vi "test_Get Slot.vi"(8 "error in (no error)":errorcluster, 11 "TestCase in":refnum<class "Scan Engine Scripting API Custom Device Unit Tests.lvclass">) -> (0 "error out":errorcluster, 3 "TestCase out":refnum<class "Scan Engine Scripting API Custom Device Unit Tests.lvclass">)   [LabVIEW 2017, in "Scan Engine Scripting API Custom Device Unit Tests.lvclass"]
uses:
  Scan Engine Scripting API Custom Device Unit Tests.lvclass
  Type Defs/Main Settings.ctl
  Type Defs/Local Chassis Settings.ctl
  Scan Engine Scripting API Custom Device Unit Tests.lvclass/Scan Engine Scripting API Custom Device Unit Tests.ctl
  186bb218-53c3-41f0-9cfc-94fa19d4683d.vi
  Utility/Set Error.vi
  <vilib>/Utility/error.llb/Clear Errors.vi
  Scripting/Modules/NI 9475/NI 9475.lvclass
  C:/dev/github.com/debryant/niveristand-scan-engine-ethercat-custom-device/Custom Device Source/Scripting/Modules/Module/Module.lvclass
  Modules.lvlibp/SD Module/SD Module.lvclass
  C:/dev/github.com/debryant/niveristand-scan-engine-ethercat-custom-device/Custom Device Source/Modules.lvlibp/RSI Module/RSI Module.lvclass
  Modules.lvlibp/RSI Module/Read Module Page Property.vi
  Modules.lvlibp/RSI Module/Read Model.vi
  Scripting/Utility/Convert Module Model to Module Class.vi
  Modules.lvlibp/SD Module/Read DIO mode.vi
  Modules.lvlibp/RSI Module/Read Channels.vi
  Scripting/Utility/Convert to DI Module.vi
  Scripting/Utility/Convert to DO Module.vi
  Scripting/Utility/Convert to CI PWM Module.vi
  Scripting/Utility/Convert to CDO Module.vi
  Scripting/Utility/Convert to PWM Module.vi
  Globals/Error Strings.vi
  Scripting/Utility/Convert to AI Vrms Module.vi
  Scripting/Utility/Convert to AI Module.vi
  Scripting/Modules/Module/Module.lvclass
  <vilib>/addons/_JKI Toolkits/VI Tester/TestCase.llb/TestCase.lvclass
  Scripting/Scan Engine Scripting.lvlib
  Scan Engine Custom Device.lvlib
  Modules/Module Test Classes/Module Test.lvclass
  C:/Program Files (x86)/National Instruments/LabVIEW 2017/vi.lib/addons/_JKI Toolkits/VI Tester/TestCase.llb/TestCase.lvclass
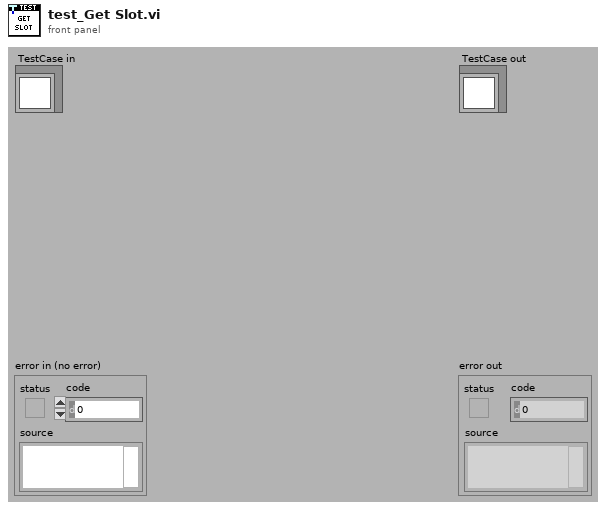
[diagram p1: front panel]
types:
  T1 = typedef "Scan Engine Custom Device.lvlib/Local Chassis Settings.ctl" = cluster{"name":string, "number of slots":i32}
  T2 = typedef "Scan Engine Custom Device.lvlib/Main Settings.ctl" = cluster{"sync to scan":bool, "scan engine decimation":u16, "delay after FPGA load (s)":u16}
  T3 = typedef "Custom Device API.lvlib/Custom Device Item Ref.ctl" = u64
  T4 = typedef "Scan Engine Scripting.lvlib/counter driven output channel settings.ctl" = cluster{"name":string, "default value":bool, "counter driven state":T5}
  T5 = typedef "Scan Engine Scripting.lvlib/Counter Driven Output Channel.lvclass/Counter Driven State.ctl" = enum16{"Disabled", "Enabled"}
  T6 = typedef "Scan Engine Scripting.lvlib/Counter Driven Output Mode.lvclass/Drive from Slot.ctl" = enum16{"Slot 1", "Slot 2", "Slot 3", "Slot 4", "Slot 5", "Slot 6", "Slot 7", "Slot 8"}
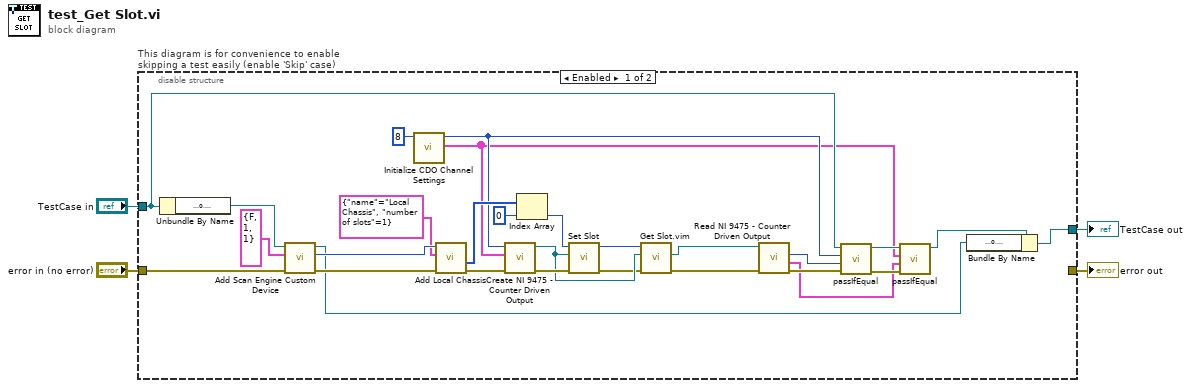
[diagram p0: block diagram]
diagram:
  n1 = disable-structure "This diagram is for convenience to enable skipping a test easily (enable 'Skip' case)" shown="Enabled" {
    disable-tunnel: "TestCase in" -> [w17 w36]
    disable-tunnel: [w21 w34] -> w1
    disable-tunnel: [_ w35] -> w3
    disable-tunnel: "error in (no error)" -> [w31 w33]
    frame Enabled {
      n2 = Unbundle By Name(w17) -> ("target ref"=w30:refnum<k24>)
      n3 = call "Add Scan Engine Custom Device.vi"("error in"=w31, "settings"=T2 {"sync to scan"=FALSE, "scan engine decimation"=1, "delay after FPGA load (s)"=1}, "target in"=w30) -> ("error out"=w29:errorcluster, "scan engine custom device ref"=w28:T3, "target out"=w9:refnum<k24>)  [unwired: 6 in]
      n4 = call "Initialize CDO Channel Settings.vi"("array size"=8) -> ("channel settings"=w12:T4[], "drive from slot"=w16:T6)  [unwired: 9 in]
      n5 = call "Add Local Chassis.vi"("error in"=w29, "settings"=T1 {"name"="Local Chassis", "number of slots"=1}, "scan engine custom device ref in"=w28) -> ("error out"=w23:errorcluster, "slot refs"=w26:T3[])  [unwired: 4 in, 3 out]
      n6 = call "Create NI 9475 - Counter Driven Output.vi"("error in"=w23, "channel settings"=w12, "drive from slot"=w16) -> ("error out"=w22:errorcluster, "NI 9475 out"=w8:refnum<class "NI 9475.lvclass">)  [unwired: 7 in]
      n7 = Index Array(array=w26, index=0) -> (element=w25:T3)
      n8 = call "Set Slot.vi"("error in"=w22, "module"=w8, "slot ref in"=w25) -> ("error out"=w5:errorcluster, "slot ref out"=w19:T3)  [unwired: 7 in]
      n9 = call "Get Slot.vim"("error in"=w5, "module in"=w8, "slot ref in"=w19) -> ("error out"=w6:errorcluster, "module"=w7:refnum<class "NI 9475.lvclass">)  [unwired: 5 in, 2 out]
      n10 = call "Read NI 9475 - Counter Driven Output.vi"("error in"=w6, "NI 9475 in"=w7) -> ("error out"=w18:errorcluster, "channel settings"=w11:T4[], "drive from slot"=w15:T6)  [unwired: 6 in, 1 out]
      n11 = call-dynamic "passIfEqual.vi"("error in (no error)"=w18, "y"=w15, "x"=w16, "TestCase in"=w17) -> ("error out"=w14:errorcluster, "TestCase out"=w13:refnum<class "Scan Engine Scripting API Custom Device Unit Tests.lvclass">)  [unwired: 6 in]
      n12 = call-dynamic "passIfEqual.vi"("error in (no error)"=w14, "y"=w11, "x"=w12, "TestCase in"=w13) -> ("TestCase out"=w10:refnum<class "Scan Engine Scripting API Custom Device Unit Tests.lvclass">)  [unwired: 6 in, 1 out]
      n13 = Bundle By Name(cluster=w10, "target ref"=w9) -> (w21:refnum<class "Scan Engine Scripting API Custom Device Unit Tests.lvclass">)
    }
    frame Disabled {
      # "skip test result while test is under development"
      n14 = call <vilib>:"skip.vi"("error in (no error)"=w33, "TestCase in"=w36) -> ("error out"=w35:errorcluster, "TestCase out"=w34:refnum<class "Scan Engine Scripting API Custom Device Unit Tests.lvclass">)  [unwired: 8 in]
    }
  }
  "error out" <- w3
  "TestCase out" <- w1
